vi "Global display 3.vi"() -> ()   [LabVIEW 2013]
panel:
  out "TEMPERATURE (N) CHART":dynamicdata(graph)
  out "TEMPERATURE (L) CHART":dynamicdata(graph)
  out "TEST VOLTS CHART":dynamicdata(graph)
  out "TEST AMPS CHART":dynamicdata(graph)
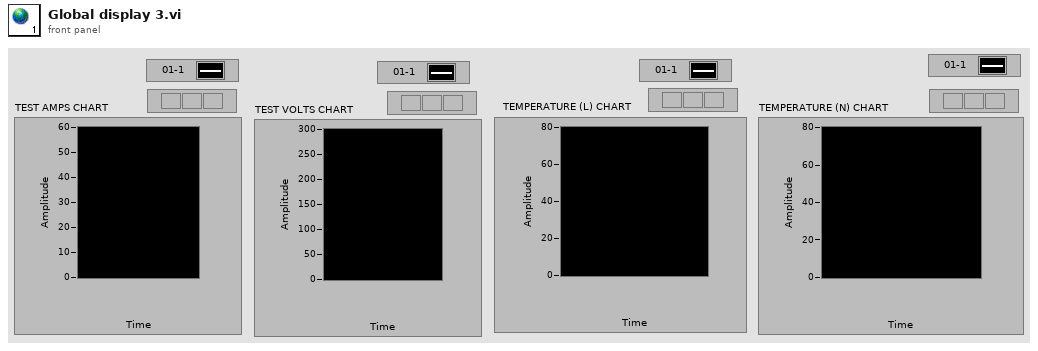
[diagram p1: front panel]
diagram:
